vi "Find in Image.vi"(2 "Template":T1(plugin-control), 4 "Image":T1(plugin-control)) -> (0 "Image Out":T1(plugin-control), 1 "Results":T2(array[cluster]) {"Score" format="%.1f"; "Position"."Y" format="%.3g"; "Position"."X" format="%.3g"})   [LabVIEW 2021]
uses:
  <vilib>/vision/NI_Vision_Development_Module.lvlib
panel:
  in  "Max # of Matches":i32=5
  in  "Minimum Score":sgl=700.0
  out "Number of Matches":i32
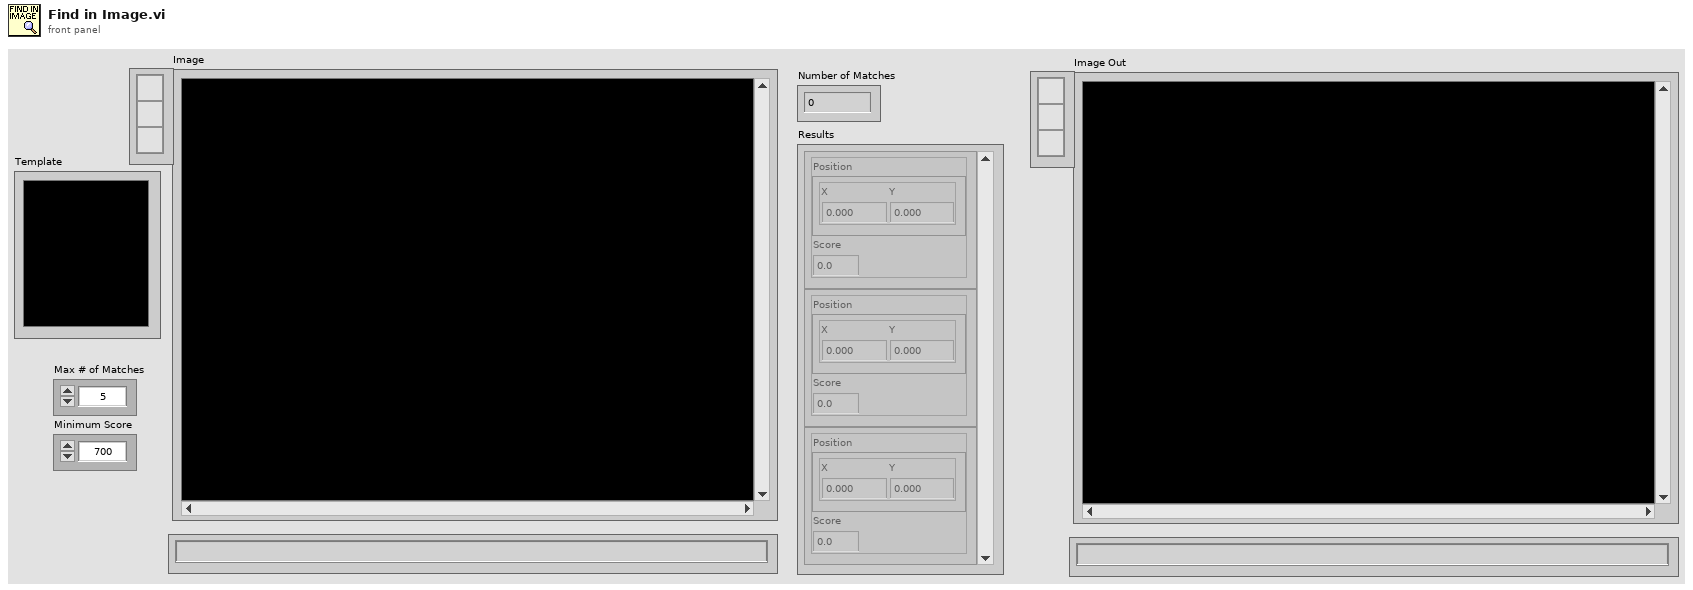
[diagram p1: front panel]
types:
  T1 = typedef "IMAQ Image.ctl" = refnum<image>
  T2 = cluster{"Position":cluster{"X":dbl, "Y":dbl}, "Score":sgl}[]
  T3 = typedef "Image Type" = u32
  T4 = cluster{"Max # of Matches":i32, "Minimum Score":sgl, "Angle Ranges":cluster{"Start Angle":sgl, "End Angle":sgl}[]}
  T5 = cluster{"Position":cluster{"x":sgl, "y":sgl}, "Angle":sgl, "Scale":sgl, "Score":sgl, "Bounding Box":cluster{"x":sgl, "y":sgl}[]}[]
  T6 = cluster{"Position":cluster{"x":sgl, "y":sgl}, "Score":sgl}
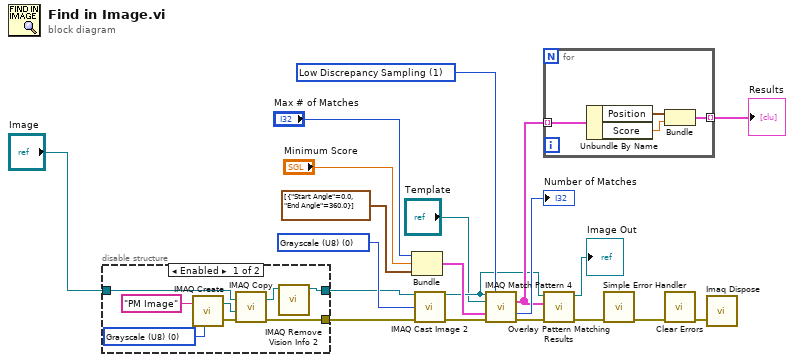
[diagram p0: block diagram]
diagram:
  w8 = T3 0 items=["Grayscale (U8)", "Grayscale (I16)", "Grayscale (SGL)", "Complex (CSG)", "RGB (U32)", "HSL (U32)", "RGB (U64)", "Grayscale (U16)"] ("Image Type")
  w9 = 1 items=["All", "Low Discrepancy Sampling", "Grayscale Value Pyramid", "Gradients Pyramid"] ("Algorithm")
  n1 = disable-structure shown="Enabled" {
    disable-tunnel: "Image" -> [w27 w29]
    disable-tunnel: [w22 w29] -> w3
    disable-tunnel: [w24 _] -> w2
    frame Enabled {
      w21 = T3 0 items=["Grayscale (U8)", "Grayscale (I16)", "Grayscale (SGL)", "Complex (CSG)", "RGB (U32)", "HSL (U32)", "RGB (U64)", "Grayscale (U16)"] ("Image Type")
      n2 = call "IMAQ Create"("Image Name"="PM Image", "Image Type"=w21) -> ("New Image"=w25:T1, "error out"=w26:errorcluster)  [unwired: 3 in]
      n3 = call "IMAQ Copy"("error in (no error)"=w26, "Image Dst"=w25, "Image Src"=w27) -> ("error out"=w24:errorcluster, "Image Dst Out"=w23:T1)  [unwired: 3 in]
      n4 = call "IMAQ Remove Vision Info 2"("Image"=w23) -> ("Image Out"=w22:T1)  [unwired: 9 in, 1 out]
    }
    frame Disabled {
    }
  }
  n5 = Bundle("Max # of Matches"="Max # of Matches", "Minimum Score"="Minimum Score", "Angle Ranges"=cluster{"Start Angle":sgl, "End Angle":sgl}[] [{"Start Angle"=0.0, "End Angle"=360.0}]) -> (w11:T4)  [unwired: 1 in]
  n6 = call "IMAQ Cast Image 2"("Image Src"=w3, "Image Type"=w8, "error in (no error)"=w2) -> ("Image Dst Out"=w7:T1, "error out"=w6:errorcluster)  [unwired: 11 in]
  n7 = call "IMAQ Match Pattern 4"("Image"=w7, "Algorithm"=w9, "Template Image"="Template", "Parameters"=w11, "error in (no error)"=w6) -> ("Matches (pixel)"=w13:T5, "Number of Matches"=→"Number of Matches":i32, "error out"=w12:errorcluster)  [unwired: 6 in, 2 out]
  n8 = for {
    tunnel: w13 -> [w33] mode=indexing
    tunnel: [w30] -> w16 mode=indexing
    n9 = Unbundle By Name(w33) -> ("Position"=w32:cluster{"x":sgl, "y":sgl}, "Score"=w31:sgl)
    n10 = Bundle("Position"=w32, "Score"=w31) -> (w30:T6)  [unwired: 1 in]
  }
  "Results" <- w16
  n11 = call "Overlay Pattern Matching Results.vi"("error in"=w12, "Matches"=w13, "Image"=w7) -> ("error out"=w14:errorcluster, "Image Out"=→"Image Out":T1)  [unwired: 7 in]
  n12 = call <vilib>:"Simple Error Handler.vi"("error in (no error)"=w14) -> ("error out"=w17:errorcluster)  [unwired: 4 in, 4 out]
  n13 = call <vilib>:"Clear Errors.vi"("error in (no error)"=w17) -> ("error out"=w20:errorcluster)  [unwired: 5 in, 1 out]
  n14 = call "Imaq Dispose"("error in (no error)"=w20) -> ()  [unwired: 5 in, 1 out]
